vi "Cockpit MS Operation.vi"() -> ()   [LabVIEW 2010]
uses:
  <vilib>/rvi/interface/nirviReadWriteControl/nirviReadWriteControl.xnode
  <vilib>/rvi/interface/nirviOpenFPGA/nirviOpenFPGA.xnode
  <vilib>/rvi/interface/nirviCloseFPGA/nirviCloseFPGA.xnode
  <vilib>/rvi/interface/nirviMethod/nirviMethod.xnode
  Subsystems/Global Variables.vi
  <vilib>/Analysis/Matrix/Datatypes/RealMatrix.ctl
  <vilib>/Analysis/Matrix/NI_Matrix.lvlib
  <vilib>/DAQmx/create/channels.llb/DAQmx Create Channel (AO-Voltage-Basic).vi
  FPGA Bitfiles/IRISSControl_FPGATarget_IRISSFPGAIOv3.3_r-h2UkgnQFc.lvbitx
  IRISS_FPGA_IO_v3.3.vi
  <vilib>/DAQmx/write.llb/DAQmx Write (Analog 1D DBL NChan 1Samp).vi
panel:
  in  "To Regulation":bool
  out "Stage PID Cluster":T1={"Stage Z PID"={"Kp"=0.0005, "Kd"=0.001, "Ki"=0.0}, "Stage Y PID"={"Kp"=0.0003, "Kd"=0.01, "Ki"=0.0}, "Stage X PID"={"Kp"=0.0003, "Kd"=0.01, "Ki"=0.0}}
  out "L1 to L4 PID Cluster":T2={"L1 PID Gains"={"Kp"=0.005, "Kd"=0.5, "Ki"=0.0005}, "L2 PID Gains"={"Kp"=0.01, "Kd"=1.0, "Ki"=0.0005}, "L3 PID Gains"={"Kp"=0.05, "Kd"=1.0, "Ki"=0.0005}, "L4 PID Gains"={"Kp"=0.1, "Kd"=1.0, "Ki"=0.0005}}
  in  "IRISS GUI":T3(tab)
  in  "Reroute Hold [sec]":dbl=10.0 caption="Hold [sec]"
  out "X Stage out [mm] 2":dbl caption="Stage X [mm]" format="%#.4f"
  out "Z Stage out [mm] 2":dbl caption="Stage Z [mm]" format="%#.4f"
  out "Y Stage out [mm] 2":dbl caption="Stage Y [mm]" format="%#.4f"
  out "Vacuum Force [mmHg]  2":i32 caption="[mmHg]"
  in  "Refractice Index":dbl=1.35
  out "Asgn Pt Out of Bound":bool caption="Assign Pt OOB"
  out "Finished Late Counts":u16
  out "Emergency alarm":bool
  out "Remote sender engaged":bool
  in  "L2 PID Gains":cluster{"Kp":dbl, "Kd":dbl, "Ki":dbl}={"Kp"=0.01, "Kd"=1.0, "Ki"=0.005}
  in  "L3 PID Gains":cluster{"Kp":dbl, "Kd":dbl, "Ki":dbl}={"Kp"=0.05, "Kd"=1.0, "Ki"=0.0005}
  in  "L4 PID Gains":cluster{"Kp":dbl, "Kd":dbl, "Ki":dbl}={"Kp"=0.1, "Kd"=0.1, "Ki"=0.0005}
  in  "L1 PID Gains":cluster{"Kp":dbl, "Kd":dbl, "Ki":dbl}={"Kp"=0.01, "Kd"=0.5, "Ki"=0.001}
  out "Current System State":T4(ring)
  out "State changing":bool
  out "Current Run No.":u8
  out "Tip out Posit":dbl[](array[numeric]) caption="Position [mm]" format="%#.3f"
  out "Tip cmd Posit":dbl[](array[numeric]) caption="Command [mm]" format="%#.3f"
  out "L4 out Posit":dbl caption="y [deg]" format="%#.2g"
  out "L4 cmd Posit":dbl caption="r [deg]" format="%#.2g"
  out "L3 out Posit":dbl caption="y [mm]" format="%#.2g"
  out "L3 cmd Posit":dbl caption="r [mm]" format="%#.2g"
  out "L2 out Posit":dbl caption="y [deg]" format="%#.2g"
  out "L2 cmd Posit":dbl caption="r [deg]" format="%#.2g"
  out "L1 out Posit":dbl caption="y [deg]" format="%#.2g"
  out "L1 cmd Posit":dbl caption="r [deg]" format="%#.2g"
  out "State Flag Array":bool[](array[boolean])
  out "Timer":i32 format="%<%M:%S>t"
  out "Irrigation Engaged? 2":bool caption="Irrigation Engaged"
  in  "Remote Control Source":u16(ring) caption="Remote Source" items=["Surgical Console", "Joystick"]
  in  "Reset Joystick":bool caption="Encoder Reset"
  out "OCT Z out [mm]":dbl caption="OCT Out Z [mm]" format="%#.4f"
  out "OCT Z cmd [mm]":dbl=6.0 caption="OCT Z Ref [mm]" min=0.0 max=12.0 step=0.5
  in  "OCT Z PID Gains":cluster{"Kp":dbl, "Kd":dbl, "Ki":dbl}={"Kp"=0.0003, "Kd"=0.0001, "Ki"=0.01}
  out "Z Stage out [mm]":dbl caption="Output Z [mm]" format="%#.4f"
  out "Z Stage cmd [mm]":dbl=6.0 caption="Reference Z [mm]" min=0.0 max=12.0 step=0.5
  out "Y Stage out [mm]":dbl caption="Output Y [mm]" format="%#.4f"
  out "Y Stage cmd [mm]":dbl=6.0 caption="Reference Y  [mm]" min=0.0 max=12.0 step=0.5
  out "X Stage out [mm]":dbl caption="Output X [mm]" format="%#.4f"
  out "X Stage cmd [mm]":dbl=6.0 caption="Reference X [mm]" min=0.0 max=12.0 step=0.5
  in  "Stage Z PID Gains":cluster{"Kp":dbl, "Kd":dbl, "Ki":dbl}={"Kp"=0.0005, "Kd"=0.001, "Ki"=0.0}
  in  "Stage Y PID Gains":cluster{"Kp":dbl, "Kd":dbl, "Ki":dbl}={"Kp"=0.0003, "Kd"=0.01, "Ki"=0.0}
  in  "Stage X PID Gains":cluster{"Kp":dbl, "Kd":dbl, "Ki":dbl}={"Kp"=0.0003, "Kd"=0.01, "Ki"=0.0}
  in  "Reroute Transit Vacf":dbl=100.0
  out "Irrigation Engaged?":bool
  in  "Z Rot Axis":dbl=1.0
  in  "Z Dist Thld":dbl[](array[numeric])=[0.5, 2.0] caption="Z Distance Threshould"
  in  "Vac Extremum":dbl[](array[numeric])=[80.0, 100.0] caption="Vacuum Extremum"
  out "Accurus Button":bool[](array[boolean]) caption="Remote Button Command"
  in  "Control: Vacuum Force":i8(slide) min=0 max=78 step=1 scale=0.0..78.0
  out "Voltage Output Ch. B":dbl(graph)
  out "Voltage Output Ch. A":dbl(graph)
  out "Accurus Engaged?":bool
  out "Vacuum Force [mmHg]":i32
  out "L4 Chart":dbl(graph) caption="L4 Waveform Chart"
  out "L3 Chart":dbl(graph) caption="L3 Waveform Chart"
  out "L2 Chart":dbl(graph) caption="L2 Waveform Chart"
  in  "Min PC Gap":dbl=0.1 caption="Min PC Gap [mm]" min=0.0 max=10.0 step=0.1 format="%#.3g"
  in  "Min AC Gap":dbl=0.1 caption="Min AC Gap [mm]" min=0.0 max=10.0 step=0.1 format="%#.3g"
  in  "Joint Limits":dbl[][](array[numeric])=[[-8.0, 35.0], [-35.0, 35.0], [-20.0, 10.0], [-40.0, 40.0]] format="%#.3g"
  in  "Offset Home 2 RCM":dbl[](array[numeric])=[-7.7, 37.0, 58.0, 0.0] format="%#.3g"
  out "Error(s) Out on Program End":errorcluster
  out "L1 Chart":dbl(graph) caption="L1 Waveform Chart"
  in  "Aiming Pt":dbl[](array[numeric])=[10.0, 0.0, -1.0, 0.0] format="%#.3g"
  in  "Engage Pt":dbl[](array[numeric])=[15.0, 0.0, 3.0, 0.0] format="%#.3g"
  in  "Inc Ctrl":dbl[](array[numeric])=[0.1, 0.05, 0.05] caption="Increment Control"
  in  "Stop Accurus":bool caption="To M/S"
  in  "L3 Go Home":bool caption="To M/S"
  in  "Program Stop":bool
  # "Robot Status"
  # "Tool Tip Location"
  # "Tracking Planning"
  # "L1"
  # "X\nY\nZ"
  # "X\nY\nZ"
  # "L2"
  # "System Progress"
  # "Assign Point Rerouting"
  # "L3"
  # "Homing finished"
  # "M/S initialization finished"
  # "Tool Cruising Boundaries"
  # "Trajecoty loading finished"
  # "XY-plane"
  # "Z-axis"
  # "Aiming finished"
  # "L4"
  # "Tool engaged"
  # "Tracking initialization finished"
  # "In Tracking"
  # "Rerouting finished"
  # "In regulation"
  # "Vacuum"
  # "X\nY"
  # "X\nY"
  # "XYZ Stage Control"
  # "OCT Z-Axis"
  # "Foot Pedal Buttons"
  # "Irrigation and Aspiration"
  # "Button 1"
  # "Button 2"
  # "Button 3"
  # "Rotation & Vacuum Force Scheduling"
  # "Joint Motion & Control"
  # "Calibration"
  # "Space Deform Parameters"
  # "L1"
  # "[deg]"
  # "S"
  # "L2"
  # "[deg]"
  # "R"
  # "[deg]"
  # "L3"
  # "[mm]"
  # "T"
  # "[mm]"
  # "L4"
  # "[deg]"
  # "First Track Point"
  # "AC & PC Gap"
  # "L1"
  # "[deg]"
  # "L2"
  # "[deg]"
  # "L3"
  # "[mm]"
  # "L4"
  # "[deg]"
  # "Error Message"
  # "Tracking Joint Limits"
  # "Incision"
  # "Min."
  # "Max."
  # "L1"
  # "L1"
  # "[deg]"
  # "L2"
  # "L2"
  # "[deg]"
  # "L3"
  # "L3"
  # "[mm]"
  # "L4"
  # "L4"
  # "[deg]"
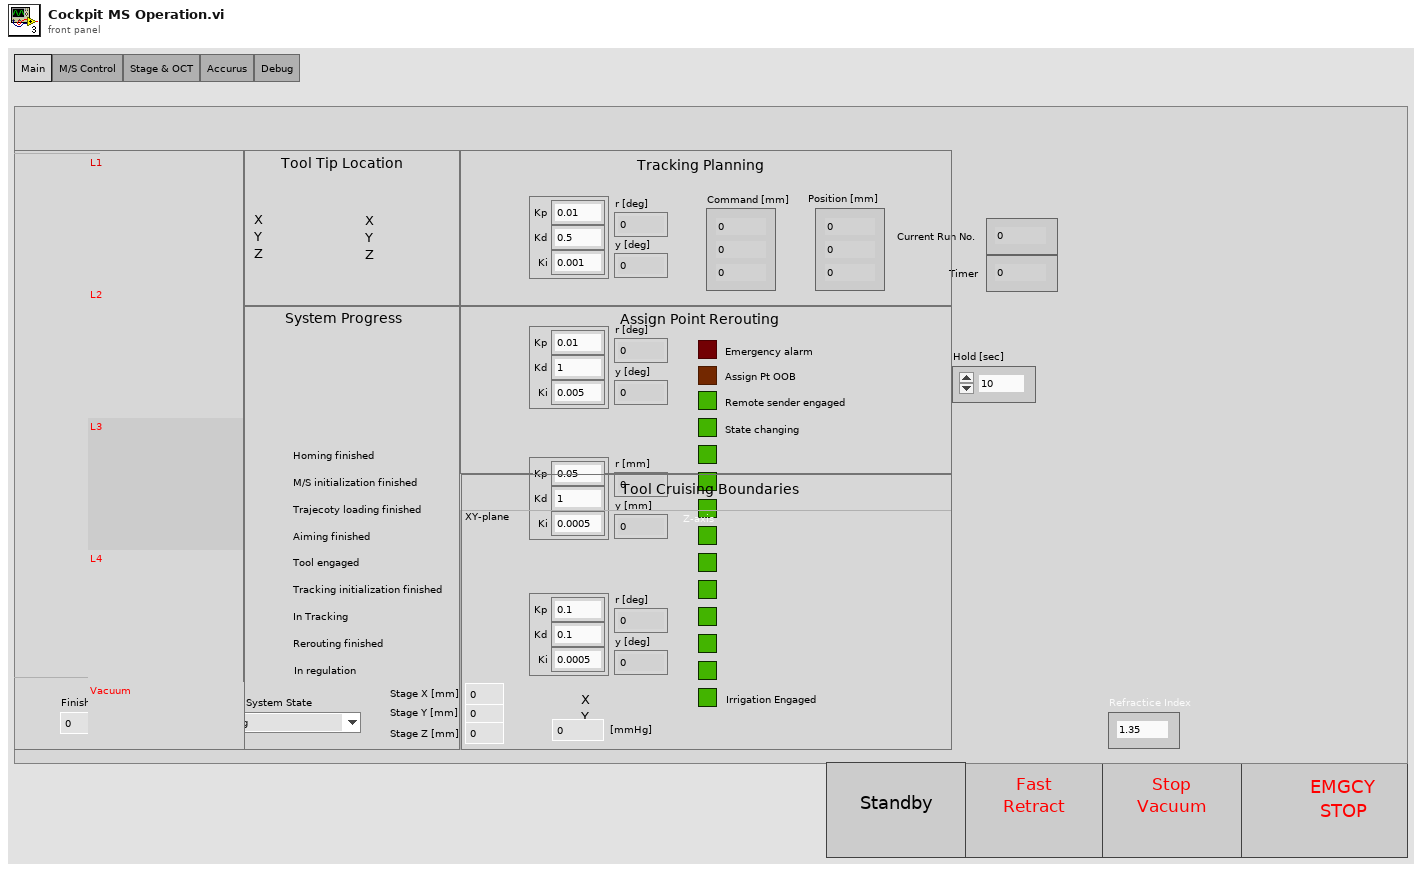
[diagram p1: front panel]
types:
  T1 = cluster{"Stage Z PID":cluster{"Kp":dbl, "Kd":dbl, "Ki":dbl}, "Stage Y PID":cluster{"Kp":dbl, "Kd":dbl, "Ki":dbl}, "Stage X PID":cluster{"Kp":dbl, "Kd":dbl, "Ki":dbl}}
  T2 = cluster{"L1 PID Gains":cluster{"Kp":dbl, "Kd":dbl, "Ki":dbl}, "L2 PID Gains":cluster{"Kp":dbl, "Kd":dbl, "Ki":dbl}, "L3 PID Gains":cluster{"Kp":dbl, "Kd":dbl, "Ki":dbl}, "L4 PID Gains":cluster{"Kp":dbl, "Kd":dbl, "Ki":dbl}}
  T3 = enum32{"Main", "M/S Control", "Stage & OCT", "Accurus", "Debug"}
  T4 = enum16{"Homing", "M/S Initialization", "M/S Operation"}
  T5 = typedef "NI_Matrix.lvlib/RealMatrix.ctl" = dbl[][]
  T6 = cluster{"X Grid":dbl[], "Y Grid":dbl[], "Za_true Surf":dbl[][], "Iris Center":dbl[], "Zp_true Surf":dbl[][], "Pinv":T5, "za_true":dbl, "za_work":dbl, "zp_work":dbl, "zp_true":dbl}
  T7 = cluster{"Traj Px Array":dbl[], "Traj Py Array":dbl[], "Traj Pz Array":dbl[], "Speed Array":dbl[], "Depth Array":dbl[]}
  T8 = cluster{"Prev L1 to L4 Posit":dbl[], "Prev Stage Posit":dbl[], "Prev OCT Z Posit":dbl}
  T9 = cluster{"L1 to L4 PID Cluster":cluster{"L1 PID Gains":cluster{"Kp":dbl, "Kd":dbl, "Ki":dbl}, "L2 PID Gains":cluster{"Kp":dbl, "Kd":dbl, "Ki":dbl}, "L3 PID Gains":cluster{"Kp":dbl, "Kd":dbl, "Ki":dbl}, "L4 PID Gains":cluster{"Kp":dbl, "Kd":dbl, "Ki":dbl}}, "Stage PID Cluster":cluster{"Stage Z PID":cluster{"Kp":dbl, "Kd":dbl, "Ki":dbl}, "Stage Y PID":cluster{"Kp":dbl, "Kd":dbl, "Ki":dbl}, "Stage X PID":cluster{"Kp":dbl, "Kd":dbl, "Ki":dbl}}, "OCT Z PID Gains":cluster{"Kp":dbl, "Kd":dbl, "Ki":dbl}}
  T10 = enum16{"Homing", "M/S Initialization", "M/S Operation", "Aiming", "Engaging", "Trajectory Loading", "Tracking Initialization", "Tracking", "Rerouting", "Regulation"}
  T11 = cluster{"Last L1 to L4 Posit":dbl[], "Last Stage Posit":dbl[], "Last OCT Z Posit":dbl}
  T12 = cluster{"Accurus button":bool[], "Accurus engaged?":bool, "Vacuum Force":i32, "Accurus Ch. A Vout":dbl, "Accurus Ch. B Vout":dbl, "Irrigation engaged?":bool}
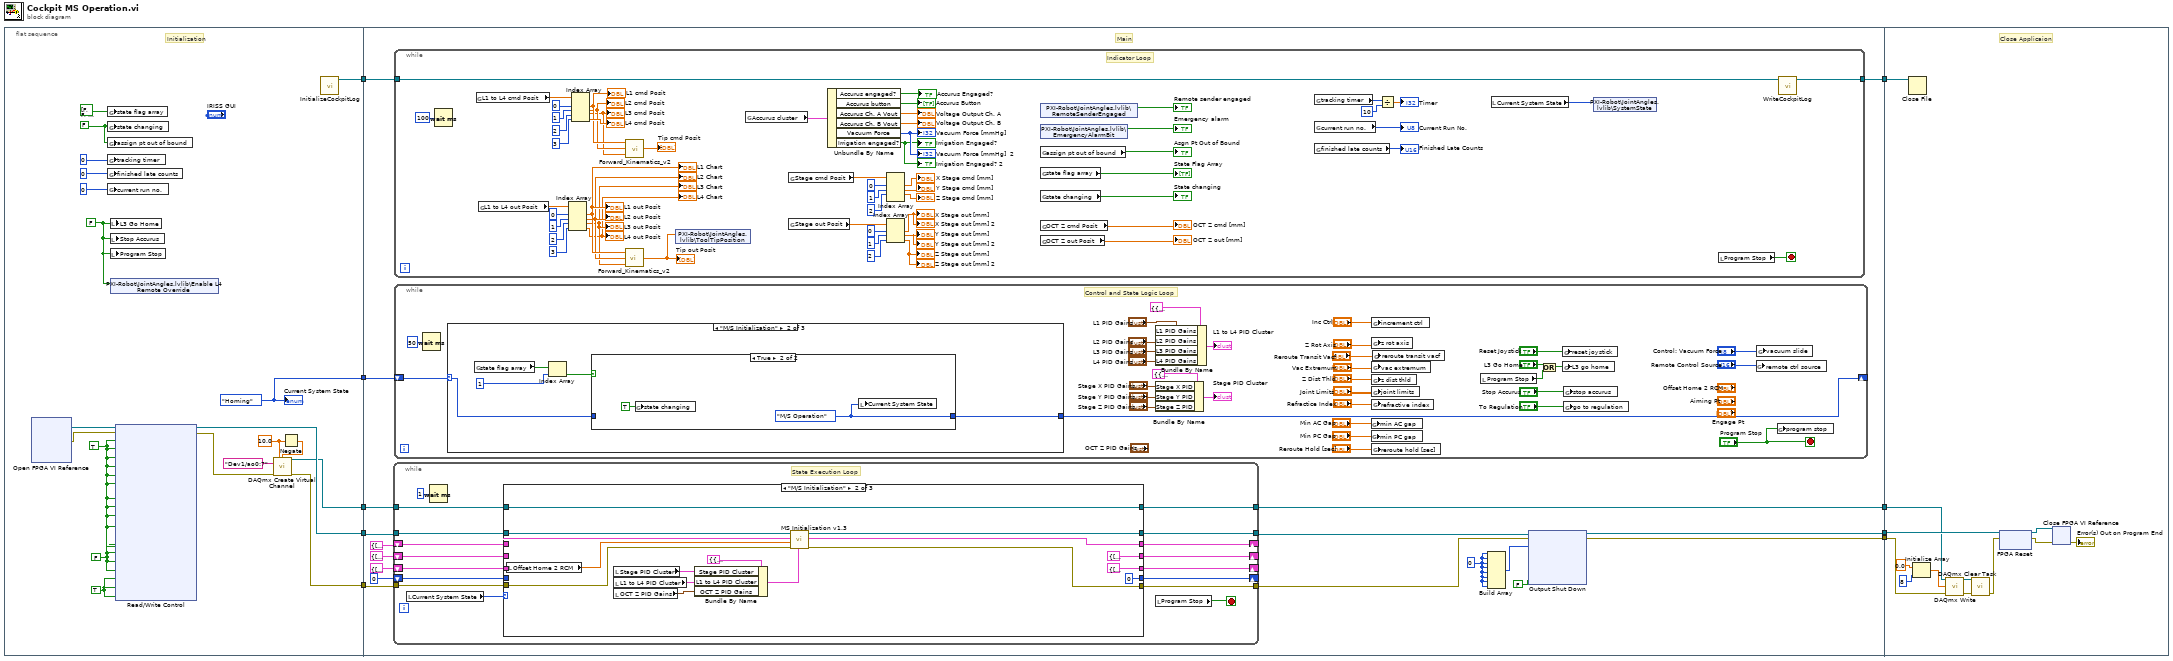
[diagram p0: block diagram]
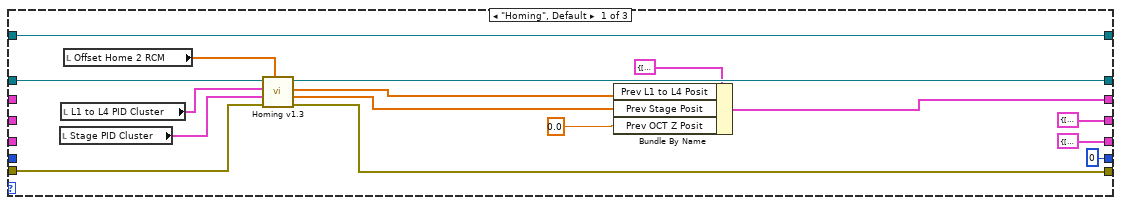
[diagram p2: hidden frame]
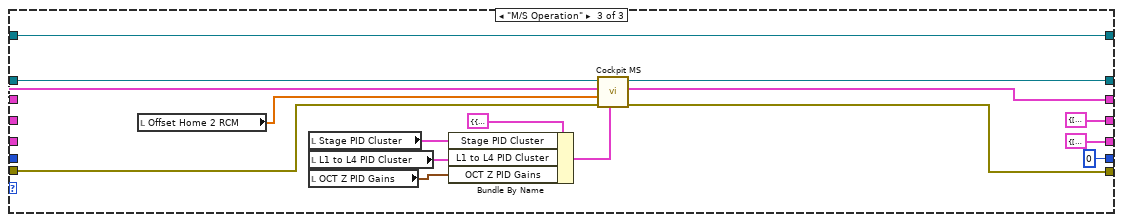
[diagram p3: hidden frame]
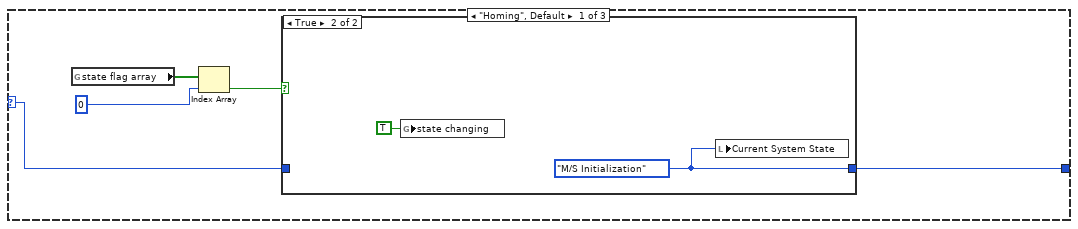
[diagram p4: hidden frame]
diagram:
  n1 = flat-sequence {
    tunnel: [w20] -> w9
    tunnel: [w19] -> w8
    tunnel: [w14] -> w7
    tunnel: [w18] -> w6
    tunnel: [w10] -> w2
    tunnel: w9 -> [w46]
    tunnel: w8 -> [w47]
    tunnel: w7 -> [w36]
    tunnel: w6 -> [w45]
    tunnel: [w39] -> w5
    tunnel: [w38] -> w4
    tunnel: [w37] -> w3
    tunnel: w2 -> [w31]
    tunnel: [w30] -> w1
    tunnel: w5 -> [w227]
    tunnel: w4 -> [w224]
    tunnel: w3 -> [w222]
    tunnel: w1 -> [w221]
    frame #0 {
      w14 = T10."Homing" ("Current State")
      w15 = FALSE ("state changing")
      w23 = 10.0
      w28 = TRUE ("Conn0/DIO12 Button 1")
      w27 = FALSE ("Reset")
      w29 = TRUE ("Reset")
      w16 = FALSE ("program stop")
      # "Initialization"
      n2 = xnode "Open FPGA VI Reference"() -> ("FPGA VI Reference Out"=w26:refnum<k20>, "error out"=w25:errorcluster)  [unwired: 2 in]
      n3 = global write "Global Variables.vi" "state flag array"(bool[] [FALSE, FALSE, FALSE, FALSE, FALSE, FALSE, FALSE, FALSE, FALSE] ("state flag array")) -> ()
      n4 = global write "Global Variables.vi" "state changing"(w15) -> ()
      n5 = global write "Global Variables.vi" "assign pt out of bound"(w15) -> ()
      n6 = global write "Global Variables.vi" "tracking timer"(0 ("finished late counts")) -> ()
      n7 = global write "Global Variables.vi" "finished late counts"(u16 0 ("finished late counts")) -> ()
      n8 = global write "Global Variables.vi" "current run no."(u8 0 ("current run no.")) -> ()
      n9 = local write "L3 Go Home"(w16) -> ()
      n10 = local write "Stop Accurus"(w16) -> ()
      n11 = local write "Program Stop"(w16) -> ()
      n12 = shared-variable "PXI-Robot\\JointAngles.lvlib\\Enable L4 Remote Override"(w16) -> ()  [unwired: 1 in, 1 out]
      n13 = xnode "Read/Write Control"("FPGA VI Reference In"=w26, "error in"=w25, "Reset 1"=w29, "Reset 3"=w29, "Reset 9"=w29, "Reset 10"=w29, "Reset 12"=w29, "Reset 13"=w29, "Reset 14"=w29, "Reset 15"=w29, "Reset 16"=w29, "Reset 17"=w29, "Reset C1-1"=w29, "Reset C1-4"=w29, "INHB X"=w27, "INHB Y"=w27, "INHB Z"=w27, "INHB OCT Mot"=w27, "Conn0/DIO12 Button 1"=w28, "Conn0/DIO13 Button 2"=w28, "Conn0/DIO15 Button 4"=w28) -> ("FPGA VI Reference Out"=w19:refnum<k20>, "error out"=w21:errorcluster)
      n14 = Negate(x=w23) -> (-x=w22:dbl)
      n15 = call-poly <vilib>:"DAQmx Create Virtual Channel.vi"("maximum value"=w23, "minimum value"=w22, "physical channels"="Dev1/ao0:7", "error in"=w21) -> ("task out"=w18:refnum<k21>, "error out"=w20:errorcluster)  [unwired: 10 in]
      n16 = call "InitializeCockpitLog.vi"() -> ("Byte Stream File out"=w10:refnum<file>)  [unwired: 11 in]
      "Current System State" <- w14
    }
    frame #1 {
      w43 = FALSE
      w34 = i16 0 ("element")
      # "Main"
      n17 = while {
        tunnel: w47 -> [w120]
        tunnel: w46 -> [w119]
        tunnel: [w118] -> w41
        tunnel: [w117] -> w40
        tunnel: w45 -> [w116]
        tunnel: [w115] -> w37
        shift-right: [w113] -> _
        shift-left: T8 {"Prev L1 to L4 Posit"=[0.0, 0.0, 0.0, 0.0], "Prev Stage Posit"=[6.0, 6.0, 6.0], "Prev OCT Z Posit"=0.0} ("Prev Posit Cluster") -> [w114]
        shift-right: [w111] -> _
        shift-left: 0 -> [w110]
        shift-right: [w109] -> _
        shift-left: T7 {"Traj Px Array"=[], "Traj Py Array"=[], "Traj Pz Array"=[], "Speed Array"=[], "Depth Array"=[]} ("Trajectory Cluster") -> [w107]
        shift-right: [w108] -> _
        shift-left: T6 {"X Grid"=[], "Y Grid"=[], "Za_true Surf"=[], "Iris Center"=[0.0, 5.0, 0.0], "Zp_true Surf"=[], "Pinv"=[[1.0, 0.0], [0.0, 1.0]], "za_true"=0.0, "za_work"=0.0, "zp_work"=0.0, "zp_true"=0.0} ("Eye Model Cluster") -> [w106]
        stop <- w112 stop-if-true
        # "State Execution Loop"
        n18 = local read "Current System State"() -> (w121:T4)
        n19 = Wait (ms)(milliseconds to wait=u32 1) -> ()  [unwired: 1 out]
        n20 = case shown="\"M/S Initialization\"" w121 {
          tunnel: w120 -> [w138 w154 w170]
          tunnel: w119 -> [w137 w153 w169]
          tunnel: [w136 w152 w168] -> w118
          tunnel: [w135 w151 w167] -> w117
          tunnel: w116 -> [w134 w150 w166]
          tunnel: [w134 w150 w166] -> w115
          tunnel: w114 -> [_ w149 w165]
          tunnel: [w133 w148 w164] -> w113
          tunnel: [0 ("Last Index") 0 ("Last Index") 0 ("Last Index")] -> w111
          tunnel: w110 -> [_ _ _]
          tunnel: [T7 {"Traj Px Array"=[], "Traj Py Array"=[], "Traj Pz Array"=[], "Speed Array"=[], "Depth Array"=[]} ("Trajectory Cluster") T7 {"Traj Px Array"=[], "Traj Py Array"=[], "Traj Pz Array"=[], "Speed Array"=[], "Depth Array"=[]} ("Trajectory Cluster") T7 {"Traj Px Array"=[], "Traj Py Array"=[], "Traj Pz Array"=[], "Speed Array"=[], "Depth Array"=[]} ("Trajectory Cluster")] -> w109
          tunnel: [T6 {"X Grid"=[], "Y Grid"=[], "Za_true Surf"=[], "Iris Center"=[0.0, 5.0, 0.0], "Zp_true Surf"=[], "Pinv"=[[1.0, 0.0], [0.0, 1.0]], "za_true"=0.0, "za_work"=0.0, "zp_work"=0.0, "zp_true"=0.0} ("Eye Model Cluster") T6 {"X Grid"=[], "Y Grid"=[], "Za_true Surf"=[], "Iris Center"=[0.0, 5.0, 0.0], "Zp_true Surf"=[], "Pinv"=[[1.0, 0.0], [0.0, 1.0]], "za_true"=0.0, "za_work"=0.0, "zp_work"=0.0, "zp_true"=0.0} ("Eye Model Cluster") T6 {"X Grid"=[], "Y Grid"=[], "Za_true Surf"=[], "Iris Center"=[0.0, 5.0, 0.0], "Zp_true Surf"=[], "Pinv"=[[1.0, 0.0], [0.0, 1.0]], "za_true"=0.0, "za_work"=0.0, "zp_work"=0.0, "zp_true"=0.0} ("Eye Model Cluster")] -> w108
          tunnel: w107 -> [_ _ _]
          tunnel: w106 -> [_ _ _]
          frame "Homing", Default {
            n21 = local read "Stage PID Cluster"() -> (w129:T1)
            n22 = local read "L1 to L4 PID Cluster"() -> (w130:T2)
            n23 = local read "Offset Home 2 RCM"() -> (w132:dbl[])
            n24 = call "Homing v1.3.vi"("Offset Home 2 RCM"=w132, "error in"=w137, "Stage PID Cluster"=w129, "L1 to L4 PID Cluster"=w130, "FPGA VI Reference In"=w138) -> ("error out"=w135:errorcluster, "Last Stage Posit"=w126:dbl[], "Last L1 to L4 Posit"=w127:dbl[], "FPGA VI Reference Out"=w136:refnum<k20>)  [unwired: 3 in]
            n25 = Bundle By Name(cluster=T8 {"Prev L1 to L4 Posit"=[-0.5409, 0.04404050915429177, -1.917656453185038, 0.02068014705882353], "Prev Stage Posit"=[6.001471972029684, 5.996134588585126, 6.000298217087839], "Prev OCT Z Posit"=-0.0} ("Prev Posit Cluster"), "Prev L1 to L4 Posit"=w127, "Prev Stage Posit"=w126, "Prev OCT Z Posit"=0.0) -> (w133:T8)
          }
          frame "M/S Initialization" {
            n26 = local read "Offset Home 2 RCM"() -> (w142:dbl[])
            n27 = local read "Stage PID Cluster"() -> (w147:T1)
            n28 = local read "L1 to L4 PID Cluster"() -> (w146:T2)
            n29 = local read "OCT Z PID Gains"() -> (w145:cluster{"Kp":dbl, "Kd":dbl, "Ki":dbl})
            n30 = Bundle By Name(cluster=T9 {"L1 to L4 PID Cluster"={"L1 PID Gains"={"Kp"=0.005, "Kd"=0.5, "Ki"=0.0005}, "L2 PID Gains"={"Kp"=0.01, "Kd"=1.0, "Ki"=0.005}, "L3 PID Gains"={"Kp"=0.05, "Kd"=1.0, "Ki"=0.0005}, "L4 PID Gains"={"Kp"=0.1, "Kd"=0.1, "Ki"=0.0005}}, "Stage PID Cluster"={"Stage Z PID"={"Kp"=0.0005, "Kd"=0.001, "Ki"=0.0}, "Stage Y PID"={"Kp"=0.0003, "Kd"=0.01, "Ki"=0.0}, "Stage X PID"={"Kp"=0.0003, "Kd"=0.01, "Ki"=0.0}}, "OCT Z PID Gains"={"Kp"=0.0003, "Kd"=0.0001, "Ki"=0.01}} ("PID Cluster"), "Stage PID Cluster"=w147, "L1 to L4 PID Cluster"=w146, "OCT Z PID Gains"=w145) -> (w143:T9)
            n31 = call "MS Initialization v1.3.vi"("PID Cluster"=w143, "error in"=w153, "Offset Home 2 RCM"=w142, "Prev Posit Cluster"=w149, "FPGA VI Reference In"=w154) -> ("error out"=w151:errorcluster, "Last Posit Cluster"=w148:T11, "FPGA VI Reference Out"=w152:refnum<k20>)  [unwired: 4 in]
          }
          frame "M/S Operation" {
            n32 = local read "Offset Home 2 RCM"() -> (w158:dbl[])
            n33 = local read "Stage PID Cluster"() -> (w163:T1)
            n34 = local read "L1 to L4 PID Cluster"() -> (w162:T2)
            n35 = local read "OCT Z PID Gains"() -> (w161:cluster{"Kp":dbl, "Kd":dbl, "Ki":dbl})
            n36 = Bundle By Name(cluster=T9 {"L1 to L4 PID Cluster"={"L1 PID Gains"={"Kp"=0.005, "Kd"=0.5, "Ki"=0.0005}, "L2 PID Gains"={"Kp"=0.01, "Kd"=1.0, "Ki"=0.005}, "L3 PID Gains"={"Kp"=0.05, "Kd"=1.0, "Ki"=0.0005}, "L4 PID Gains"={"Kp"=0.1, "Kd"=0.1, "Ki"=0.0005}}, "Stage PID Cluster"={"Stage Z PID"={"Kp"=0.0005, "Kd"=0.001, "Ki"=0.0}, "Stage Y PID"={"Kp"=0.0003, "Kd"=0.01, "Ki"=0.0}, "Stage X PID"={"Kp"=0.0003, "Kd"=0.01, "Ki"=0.0}}, "OCT Z PID Gains"={"Kp"=0.0003, "Kd"=0.0001, "Ki"=0.01}} ("PID Cluster"), "Stage PID Cluster"=w163, "L1 to L4 PID Cluster"=w162, "OCT Z PID Gains"=w161) -> (w159:T9)
            n37 = call "Cockpit MS.vi"("PID Cluster"=w159, "error in"=w169, "Offset Home 2 RCM"=w158, "Prev Posit Cluster"=w165, "FPGA VI Reference In"=w170) -> ("error out"=w167:errorcluster, "Last Posit Cluster"=w164:T11, "FPGA VI Reference Out"=w168:refnum<k20>)  [unwired: 4 in]
          }
        }
        n38 = local read "Program Stop"() -> (w112:bool)
      }
      n39 = while {
        shift-right: [w178] -> _
        shift-left: w36 -> [w179]
        stop <- "Program Stop" stop-if-true
        # "Control and State Logic Loop"
        n40 = Wait (ms)(milliseconds to wait=u32 50) -> ()  [unwired: 1 out]
        n41 = case shown="\"M/S Initialization\"" w179 {
          selector: w179 -> [w206 w212 w220]
          tunnel: [w205 w213 w220] -> w178
          frame "Homing", Default {
            n42 = global read "Global Variables.vi" "state flag array"() -> (w207:bool[])
            n43 = Index Array(array=w207, index=0) -> (element=w204:bool)
            n44 = case shown="True" w204 {
              tunnel: [w209 w210] -> w205
              tunnel: w206 -> [w209 _]
              frame False {
                # "homing in process"
              }
              frame True {
                w210 = T10."M/S Initialization" ("Current State")
                # "finish homing"
                n45 = global write "Global Variables.vi" "state changing"(TRUE ("state changing")) -> ()
                n46 = local write "Current System State"(w210) -> ()
              }
            }
          }
          frame "M/S Initialization" {
            n47 = global read "Global Variables.vi" "state flag array"() -> (w215:bool[])
            n48 = Index Array(array=w215, index=1) -> (element=w214:bool)
            n49 = case shown="True" w214 {
              tunnel: [w217 w218] -> w213
              tunnel: w212 -> [w217 _]
              frame False {
              }
              frame True {
                w218 = T10."M/S Operation" ("Current State")
                n50 = global write "Global Variables.vi" "state changing"(TRUE ("state changing")) -> ()
                n51 = local write "Current System State"(w218) -> ()
              }
            }
          }
          frame "M/S Operation" {
          }
        }
        n52 = Bundle By Name(cluster=T2 {"L1 PID Gains"={"Kp"=0.005, "Kd"=0.5, "Ki"=0.0005}, "L2 PID Gains"={"Kp"=0.01, "Kd"=1.0, "Ki"=0.0005}, "L3 PID Gains"={"Kp"=0.05, "Kd"=1.0, "Ki"=0.0005}, "L4 PID Gains"={"Kp"=0.1, "Kd"=1.0, "Ki"=0.0005}} ("L1 to L4 PID Cluster 2"), "L1 PID Gains"="L1 PID Gains", "L2 PID Gains"="L2 PID Gains", "L3 PID Gains"="L3 PID Gains", "L4 PID Gains"="L4 PID Gains") -> (→"L1 to L4 PID Cluster":T2)
        n53 = Bundle By Name(cluster=T1 {"Stage Z PID"={"Kp"=0.0005, "Kd"=0.001, "Ki"=0.0}, "Stage Y PID"={"Kp"=0.0003, "Kd"=0.01, "Ki"=0.0}, "Stage X PID"={"Kp"=0.0003, "Kd"=0.01, "Ki"=0.0}} ("Stage PID Cluster 2"), "Stage X PID"="Stage X PID Gains", "Stage Y PID"="Stage Y PID Gains", "Stage Z PID"="Stage Z PID Gains") -> (→"Stage PID Cluster":T1)
        n54 = global write "Global Variables.vi" "min AC gap"("Min AC Gap") -> ()
        n55 = global write "Global Variables.vi" "min PC gap"("Min PC Gap") -> ()
        n56 = global write "Global Variables.vi" "increment ctrl"("Inc Ctrl") -> ()
        n57 = global write "Global Variables.vi" "z rot axis"("Z Rot Axis") -> ()
        n58 = global write "Global Variables.vi" "vac extremum"("Vac Extremum") -> ()
        n59 = global write "Global Variables.vi" "z dist thld"("Z Dist Thld") -> ()
        n60 = global write "Global Variables.vi" "joint limits"("Joint Limits") -> ()
        n61 = global write "Global Variables.vi" "refractive index"("Refractice Index") -> ()
        n62 = global write "Global Variables.vi" "reroute hold [sec]"("Reroute Hold [sec]") -> ()
        n63 = global write "Global Variables.vi" "reroute transit vacf"("Reroute Transit Vacf") -> ()
        n64 = local read "Program Stop"() -> (w182:bool)
        n65 = Or(x="L3 Go Home", y=w182) -> (x .or. y?=w183:bool)
        n66 = global write "Global Variables.vi" "reset joystick"("Reset Joystick") -> ()
        n67 = global write "Global Variables.vi" "L3 go home"(w183) -> ()
        n68 = global write "Global Variables.vi" "stop accurus"("Stop Accurus") -> ()
        n69 = global write "Global Variables.vi" "go to regulation"("To Regulation") -> ()
        n70 = global write "Global Variables.vi" "remote ctrl source"("Remote Control Source") -> ()
        n71 = global write "Global Variables.vi" "vacuum slide"("Control: Vacuum Force") -> ()
        n72 = global write "Global Variables.vi" "program stop"("Program Stop") -> ()
      }
      n73 = while {
        tunnel: w31 -> [w49]
        tunnel: [w48] -> w30
        stop <- w86 stop-if-true
        # "Indicator Loop"
        n74 = Wait (ms)(milliseconds to wait=u32 100) -> ()  [unwired: 1 out]
        n75 = global read "Global Variables.vi" "L1 to L4 cmd Posit"() -> (w78:dbl[])
        n76 = global read "Global Variables.vi" "L1 to L4 out Posit"() -> (w81:dbl[])
        n77 = Index Array(array=w81, index #1=0 ("index"), index #2=1 ("index"), index #3=2 ("index"), index #4=3 ("index")) -> (element #1=w53:dbl, element #2=w52:dbl, element #3=w51:dbl, element #4=→"L4 out Posit" →"L4 Chart":dbl)
        "L3 out Posit" <- w51
        "L2 out Posit" <- w52
        "L1 out Posit" <- w53
        "L1 Chart" <- w53
        "L2 Chart" <- w52
        "L3 Chart" <- w51
        n78 = Index Array(array=w78, index #1=0 ("index"), index #2=1 ("index"), index #3=2 ("index"), index #4=3 ("index")) -> (element #1=w85:dbl, element #2=w84:dbl, element #3=w83:dbl, element #4=→"L4 cmd Posit":dbl)
        "L1 cmd Posit" <- w85
        "L3 cmd Posit" <- w83
        "L2 cmd Posit" <- w84
        n79 = call "Forward_Kinematics_v2.vi"("theta 3"=w51, "theta 2"=w52, "theta 1"=w53) -> ("position"=w73:dbl[])
        "Tip out Posit" <- w73
        n80 = call "Forward_Kinematics_v2.vi"("theta 3"=w83, "theta 2"=w84, "theta 1"=w85) -> ("position"=→"Tip cmd Posit":dbl[])
        n81 = shared-variable "PXI-Robot\\JointAngles.lvlib\\ToolTipPosition"(w73) -> ()  [unwired: 1 in, 1 out]
        n82 = global read "Global Variables.vi" "Accurus cluster"() -> (w67:T12)
        n83 = global read "Global Variables.vi" "Stage cmd Posit"() -> (w79:dbl[])
        n84 = global read "Global Variables.vi" "Stage out Posit"() -> (w80:dbl[])
        n85 = Unbundle By Name(w67) -> ("Accurus engaged?"=→"Accurus Engaged?":bool, "Accurus button"=→"Accurus Button":bool[], "Accurus Ch. A Vout"=→"Voltage Output Ch. A":dbl, "Accurus Ch. B Vout"=→"Voltage Output Ch. B":dbl, "Vacuum Force"=→"Vacuum Force [mmHg]" →"Vacuum Force [mmHg]  2":i32, "Irrigation engaged?"=→"Irrigation Engaged?" →"Irrigation Engaged? 2":bool)
        n86 = Index Array(array=w80, index #1=0 ("index"), index #2=1 ("index"), index #3=2 ("index")) -> (element #1=→"X Stage out [mm]" →"X Stage out [mm] 2":dbl, element #2=→"Y Stage out [mm]" →"Y Stage out [mm] 2":dbl, element #3=→"Z Stage out [mm]" →"Z Stage out [mm] 2":dbl)
        n87 = Index Array(array=w79, index #1=0 ("index"), index #2=1 ("index"), index #3=2 ("index")) -> (element #1=→"X Stage cmd [mm]":dbl, element #2=→"Y Stage cmd [mm]":dbl, element #3=→"Z Stage cmd [mm]":dbl)  [unwired: 1 in, 1 out]
        n88 = shared-variable "PXI-Robot\\JointAngles.lvlib\\RemoteSenderEngaged"() -> (→"Remote sender engaged":bool)  [unwired: 1 in, 1 out]
        n89 = shared-variable "PXI-Robot\\JointAngles.lvlib\\EmergencyAlarmBit"() -> (→"Emergency alarm":bool)  [unwired: 1 in, 1 out]
        n90 = global read "Global Variables.vi" "assign pt out of bound"() -> (→"Asgn Pt Out of Bound":bool)
        n91 = global read "Global Variables.vi" "state flag array"() -> (→"State Flag Array":bool[])
        n92 = global read "Global Variables.vi" "state changing"() -> (→"State changing":bool)
        n93 = global read "Global Variables.vi" "OCT Z cmd Posit"() -> (→"OCT Z cmd [mm]":dbl)
        n94 = global read "Global Variables.vi" "OCT Z out Posit"() -> (→"OCT Z out [mm]":dbl)
        n95 = global read "Global Variables.vi" "tracking timer"() -> (w62:i32)
        n96 = global read "Global Variables.vi" "current run no."() -> (→"Current Run No.":u8)
        n97 = global read "Global Variables.vi" "finished late counts"() -> (→"Finished Late Counts":u16)
        n98 = Divide(x=w62, y=10) -> (x/y=→"Timer":dbl)
        n99 = local read "Current System State"() -> (w54:T4)
        n100 = shared-variable "PXI-Robot\\JointAngles.lvlib\\SystemState"(w54) -> ()  [unwired: 1 in, 1 out]
        n101 = local read "Program Stop"() -> (w86:bool)
        n102 = call "WriteCockpitLog.vi"("File In"=w49) -> ("File Out"=w48:refnum<file>)  [unwired: 10 in]
      }
      n103 = Build Array(w34, w34, w34, w34, w34, w34, w34, w34) -> (w42:i16[])
      n104 = xnode "Output Shut Down"("FPGA VI Reference In"=w41, "error in"=w40, "AO"=w42, "INHB X"=w43, "INHB Y"=w43, "INHB Z"=w43, "INHB OCT Mot"=w43) -> ("FPGA VI Reference Out"=w38:refnum<k20>, "error out"=w39:errorcluster)
    }
    frame #2 {
      # "Close Applicaion"
      n105 = Close File(refnum=w221) -> ()  [unwired: 1 in, 2 out]
      n106 = Initialize Array(0.0 ("element"), 8 ("dimension size")) -> (w228:dbl[])
      n107 = call-poly <vilib>:"DAQmx Write.vi"("task/channels in"=w222, "data"=w228, "error in"=w227) -> ("task out"=w226:refnum<k21>, "error out"=w225:errorcluster)  [unwired: 10 in, 1 out]
      n108 = call <vilib>:"DAQmx Clear Task.vi"("task in"=w226, "error in"=w225) -> ("error out"=w223:errorcluster)  [unwired: 13 in]
      n109 = xnode "FPGA Reset"("FPGA VI Reference In"=w224, "error in"=w223) -> ("FPGA VI Reference Out"=w233:refnum<k20>, "error out"=w232:errorcluster)
      n110 = xnode "Close FPGA VI Reference"("FPGA VI Reference In"=w233, "error in"=w232) -> ("error out"=→"Error(s) Out on Program End":errorcluster)
    }
  }
